vi "Init.vi"(7 "Lumberjack.lvlib:Layout.lvclass":refnum<class "Layout.lvclass">, 8 "error in (no error)":errorcluster, 10 "FileAppenderConfig":T1={"common"={"id"="", "threshold"=enum."INFO", "filter"={"mode"=enum."Mirror", "levelMin"=enum."INFO", "levelMax"=enum."INFO", "tagPrefix"=""}, "queueBound"=0, "dropPolicy"=enum."DropOldest", "useUTC"=FALSE}, "file"={"rootFolder"=path "", "maxFileSize"=0, "maxFileCount"=0, "baseName"="", "extension"="", "delimiter"="", "calendarFolderTree"=FALSE}}, 11 "FileAppender in":refnum<class "FileAppender.lvclass">) -> (0 "error out":errorcluster, 3 "FileAppender out":refnum<class "FileAppender.lvclass">)   [LabVIEW 2026, in "Lumberjack.lvlib" / "FileAppender.lvclass"]
uses:
  FileAppender.lvclass
  C:/Users/dallis/OneDrive - Velico Medical/Documents/Personal/LabVIEW Coding Projects/Lumberjack/src/Core/Appenders/Appender.lvclass/Appender.lvclass
  Layouts/Layout.lvclass/Layout.lvclass
  TypeDefs/FileAppenderConfig.ctl
  TypeDefs/AppenderConfig.ctl
  TypeDefs/Severity.ctl
  TypeDefs/Filter.ctl
  TypeDefs/FilterMode.ctl
  TypeDefs/DropPolicy.ctl
  TypeDefs/FileConfig.ctl
  FileAppender.lvclass/FileAppender.ctl
  Layouts/Layout.lvclass/Write useUTC.vi
  Appender.lvclass/Appender.lvclass
  Lumberjack.lvlib
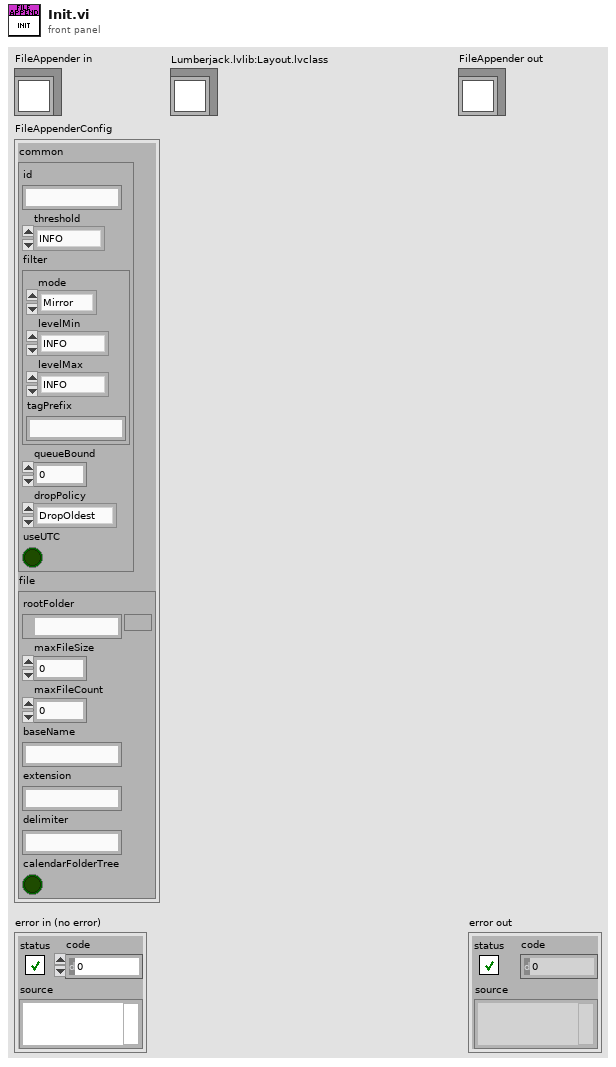
[diagram p1: front panel]
types:
  T1 = typedef "Lumberjack.lvlib/FileAppenderConfig.ctl" = cluster{"common":T2, "file":T7}
  T2 = typedef "Lumberjack.lvlib/AppenderConfig.ctl" = cluster{"id":string, "threshold":T3, "filter":T4, "queueBound":i32, "dropPolicy":T6, "useUTC":bool}
  T3 = typedef "Lumberjack.lvlib/Severity.ctl" = enum16{"OFF", "FATAL", "ERROR", "WARN", "INFO", "DEBUG", "TRACE", "ALL"}
  T4 = typedef "Lumberjack.lvlib/Filter.ctl" = cluster{"mode":T5, "levelMin":T3, "levelMax":T3, "tagPrefix":string}
  T5 = typedef "Lumberjack.lvlib/FilterMode.ctl" = enum16{"Mirror", "Routed"}
  T6 = typedef "Lumberjack.lvlib/DropPolicy.ctl" = enum16{"DropOldest", "DropNewest", "LevelAware"}
  T7 = typedef "Lumberjack.lvlib/FileConfig.ctl" = cluster{"rootFolder":path, "maxFileSize":i64, "maxFileCount":i32, "baseName":string, "extension":string, "delimiter":string, "calendarFolderTree":bool}
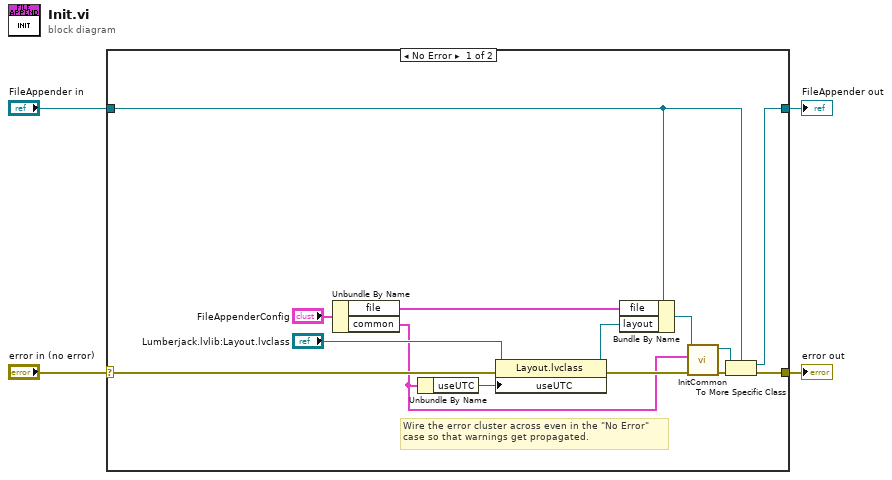
[diagram p0: block diagram]
diagram:
  n1 = case shown="No Error" "error in (no error)" {
    selector: "error in (no error)" -> [w16 w20]
    tunnel: [w11 w20] -> w3
    tunnel: [w8 w19] -> w1
    tunnel: "FileAppender in" -> [w10 w19]
    frame No Error {
      # "Wire the error cluster across even in the \"No Error\"\ncase so that warnings get propagated."
      n2 = Unbundle By Name("FileAppenderConfig") -> ("file"=w6:T7, "common"=w5:T2)
      n3 = Unbundle By Name(w5) -> ("useUTC"=w17:bool)
      n4 = property class="Layout.lvclass"(reference="Lumberjack.lvlib:Layout.lvclass", error in=w16, "useUTC"=w17) -> (reference out=w18:refnum<class "Layout.lvclass">, error out=w15:errorcluster)
      n5 = Bundle By Name(cluster=w10, "file"=w6, "layout"=w18) -> (w13:refnum<class "FileAppender.lvclass">)
      n6 = call "InitCommon.vi"("error in (no error)"=w15, "AppenderConfig"=w5, "Appender in"=w13) -> ("error out"=w12:errorcluster, "Appender out"=w9:refnum<class "FileAppender.lvclass">)  [unwired: 7 in]
      n7 = To More Specific Class(target class=w10, reference=w9, error in=w12) -> (specific class reference=w8:refnum<class "FileAppender.lvclass">, error out=w11:errorcluster)
    }
    frame Error {
    }
  }
  "error out" <- w3
  "FileAppender out" <- w1
